vi "Build Modified.vi"(9 "index":i32, 10 "build modified":T1={"App Name"="", "Build Type"=enum."Fix", "Current Version"="", "Next Version"="", "Check"=FALSE}, 11 "GUI Builder in":refnum<class "GUI Builder.lvclass">) -> (3 "GUI Builder out":refnum<class "GUI Builder.lvclass">)   [LabVIEW 2021, in "App-Builder Library.lvlib" / "GUI Builder.lvclass"]
uses:
  GUI Builder.lvclass
  Builder/Builder.lvclass
  Builder/Build Type.ctl
  Builder/App descriptions.ctl
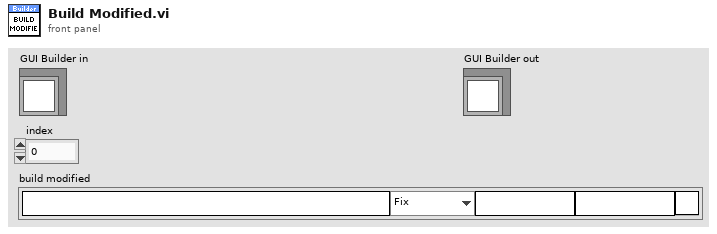
[diagram p1: front panel]
types:
  T1 = typedef "App-Builder Library.lvlib/Builder.lvclass/App descriptions.ctl" = cluster{"App Name":string, "Build Type":T2, "Current Version":string, "Next Version":string, "Check":bool}
  T2 = typedef "App-Builder Library.lvlib/Builder.lvclass/Build Type.ctl" = enum16{"Major", "Minor", "Fix", "Build"}
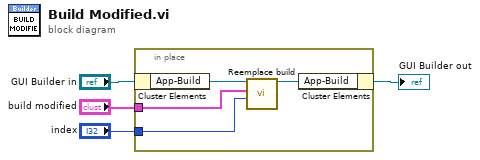
[diagram p0: block diagram]
diagram:
  n1 = in-place {
    in-place-border: "build modified" -> [w8]
    in-place-border: "index" -> [w7]
    n2 = in-place-cluster #1("GUI Builder in") -> ("App-Build"=w5:refnum<class "Builder.lvclass">)
    n3 = call "Reemplace build.vi"("index"=w7, "build modified"=w8, "Builder in"=w5) -> ("Builder out"=w6:refnum<class "Builder.lvclass">)  [unwired: 8 in]
    n4 = in-place-cluster #1("App-Build"=w6) -> (→"GUI Builder out":refnum<class "GUI Builder.lvclass">)
  }
